vi "Single Slow IV v1.6.vi"() -> ()   [LabVIEW 2020]
uses:
  <vilib>/Utility/file.llb/Write Delimited Spreadsheet (DBL).vi
panel:
  out "DAQ_AI_Reader endpoint":refnum<k21>
  out "DAQ_CMD_Writer endpoint":refnum<k21>
  out "Current variable":dbl=2.9
  in  "stop":bool
  in  "Tab Control 2":T1(tab)=enum."PID"
  out "cRIO data plot":cluster{"Y":dbl[], "Y":dbl[]}[](graph)
  out "cRIO Plot 0":string="DC Voltage V"
  out "cRIO Plot 1":string="DC current uA"
  out "cRIO Plot 2":string="dV V"
  out "cRIO Plot 3":string="dI uA"
  out "Lockin X":cluster{"Y":dbl[], "Y":dbl[]}[](graph)
  out "Lockin Y":cluster{"Y":dbl[], "Y":dbl[]}[](graph)
  in  "Tab Control":T2(tab)
  out "Unit":string="uA"
  in  "Tab for variable":enum32{"Current", "Magnetic field"}(tab)=enum."Magnetic field"
  in  "Delay Time s":dbl=11.0 caption="Delay Time (s)"
  in  "AO Channel":string(combo)="AO0"
  in  "current output Scale factor":dbl=1.0
  in  "Fixed current uA":dbl=2.1
  in  "Scale factor":dbl=1.0
  in  "Field Rate mT per sec":dbl=0.1 format="%#_13g"
  in  "Magnet Device Select":string(combo)="NI DAQ Controlled V to I source"
  in  "Start":dbl=1.4
  in  "Range":dbl=1.5
  in  "Step":dbl=0.005
  in  "Ramp type":string(combo)="Range"
  in  "Ramp up first T":bool=TRUE
  in  "cRIO Chan 0":bool=TRUE
  in  "cRIO IP":string="//172.22.11.2"
  in  "Reading Average times":i32=20
  in  "read cRIO":bool=TRUE
  in  "Scale factor3":dbl=1.0
  in  "Channel name 3":string(combo)="dI uA"
  in  "cRIO Chan 3":bool
  in  "Scale factor2":dbl=1.0
  in  "Channel name 2":string(combo)="dV V"
  in  "cRIO Chan 2":bool
  in  "Scale factor1":dbl=1.0
  in  "Channel name 1":string(combo)="DC current uA"
  in  "cRIO Chan 1":bool=TRUE
  in  "Scale factor0":dbl=0.0001
  in  "Channel name 0":string(combo)="DC Voltage V"
  in  "Lockin address 4":string
  in  "Lockin address 3":string
  in  "Lockin address 2":string="GPIB0::9::INSTR"
  in  "Lockin address 1":string="GPIB0::8::INSTR"
  in  "Lockin 4":bool
  in  "Lockin 3":bool
  in  "Lockin 2":bool=TRUE
  in  "Lockin 1":bool=TRUE
  in  "Use Lockin":bool=TRUE
  in  "Lockin Chan name 4":string(combo)="None"
  in  "Lockin Chan name 3":string(combo)="None"
  in  "Lockin Chan name 2":string(combo)="Current mV"
  in  "Lockin Chan name 1":string(combo)="Voltage mV"
  in  "Lockin and field and temperature status":string="Data File time stamp 20210729-111405\nTemperature Chan1 1.218210, Chan2 0.050001\nmagnetic field InfmT\nLockin status\n#Device channel name Voltage mV#Device \u0000\u0000\u0000\u000fGPIB0::8::INSTR\n #PHASE=0\n #REF=1\n #FREQ=197\n #INPUT=0\n #SENS=24\n #TIMECONST=12\n #VOLTAGE=0.1\n#Device channel name Current mV#Device \u0000\u0000\u0000\u000fGPIB0::9::INSTR\n #PHASE=0\n #REF=0\n #FREQ=196.996\n #INPUT=0\n #SENS=22\n #TIMECONST=10\n #VOLTAGE=0.004\n"
  in  "Temp Device":string(combo)="Elsa"
  in  "Temp Chan1":string="T5"
  in  "Temp Chan2":string="T8"
  in  "Magnetic field read device":string(combo)="Elsa Magnet"
  in  "Record Field":bool
  in  "Contour plot folder":path=path "C:/Users/gyue/Desktop/Data folder 20210720"
  out "error out":errorcluster
  # "Voltage x factor=uA"
  # "Voltage x factor=uA"
  # "Voltage x factor=actual"
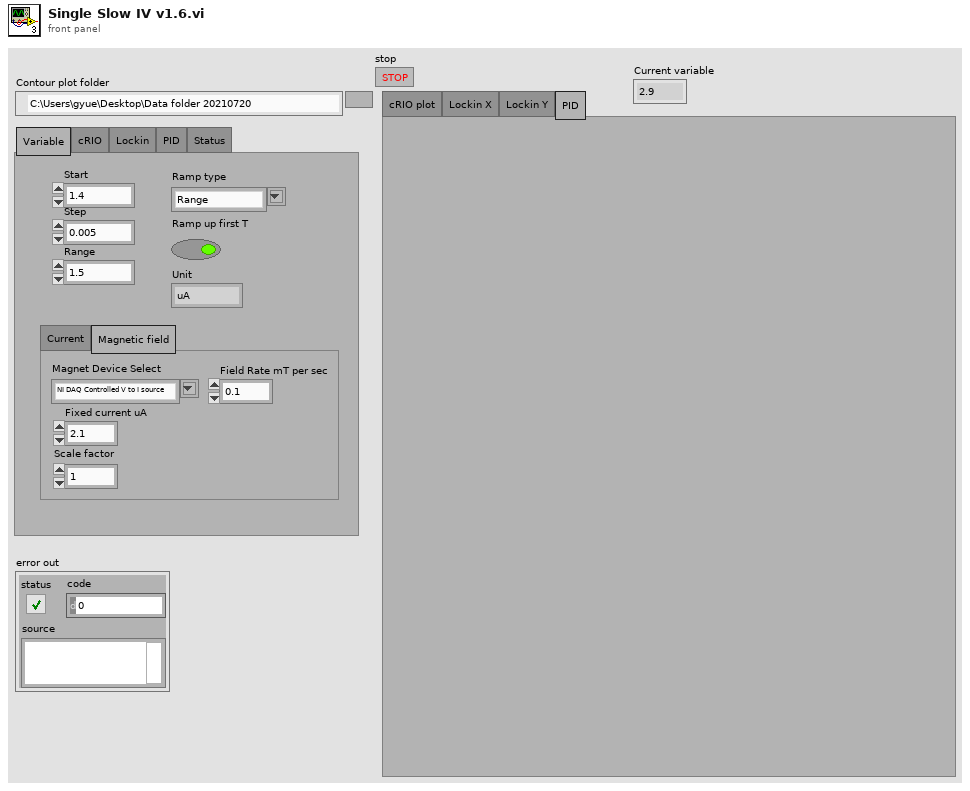
[diagram p1: front panel]
types:
  T1 = enum32{"cRIO plot", "Lockin X", "Lockin Y", "PID"}
  T2 = enum32{"Variable", "cRIO", "Lockin", "PID", "Status"}
  T3 = cluster{"AI0":dbl, "AI1":dbl, "AI2":dbl, "AI3":dbl}
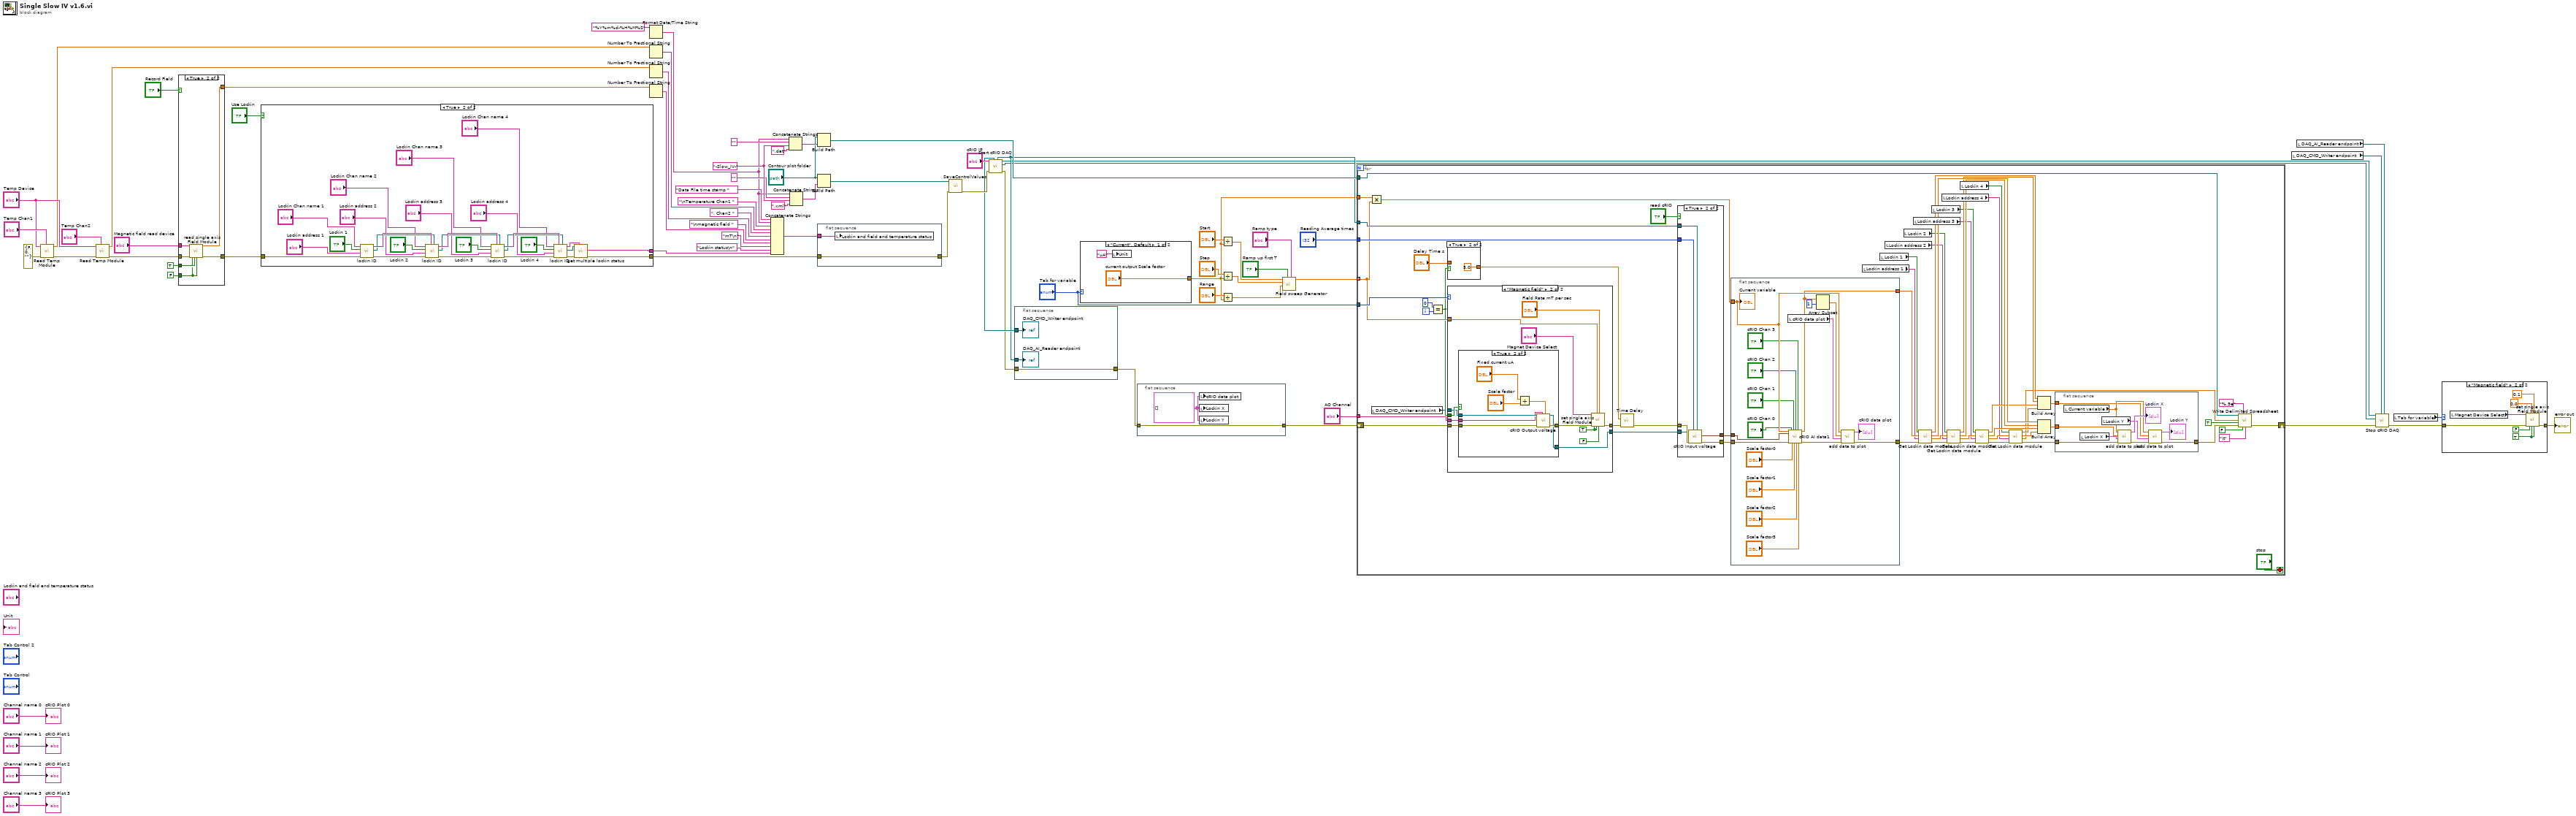
[diagram p0: block diagram]
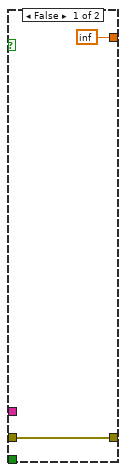
[diagram p2: hidden frame]
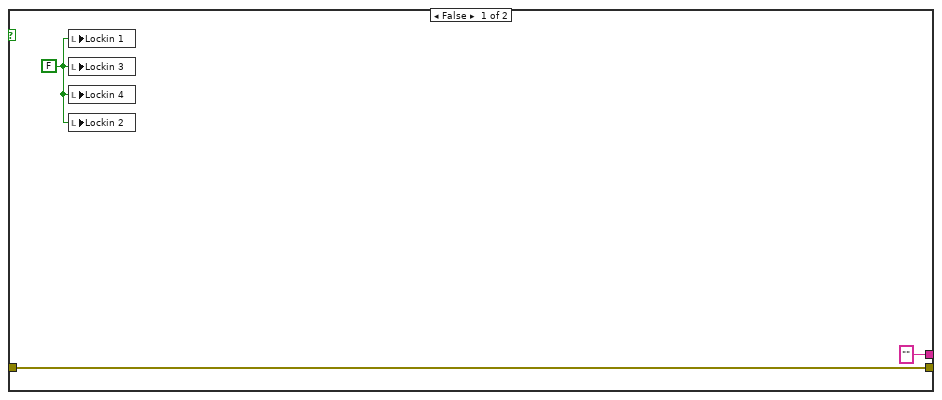
[diagram p3: hidden frame]
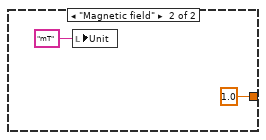
[diagram p5: hidden frame]
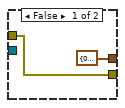
[diagram p6: hidden frame]
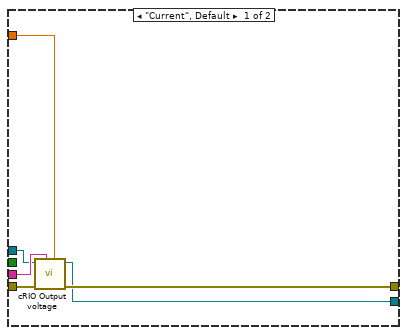
[diagram p7: hidden frame]
diagram:
  w66 = "-Slow_IV-"
  n1 = call "Read Temp Module.vi"("Temp Chan"="Temp Chan1", "error in (no error)"=errorcluster {"status"=FALSE, "code"=0, "source"=""} ("error in"), "Device"="Temp Device") -> ("error out"=w36:errorcluster, "Temperature K"=w31:dbl)  [unwired: 7 in]
  n2 = call "Read Temp Module.vi"("Temp Chan"="Temp Chan2", "error in (no error)"=w36, "Device"="Temp Device") -> ("error out"=w29:errorcluster, "Temperature K"=w30:dbl)  [unwired: 7 in]
  n3 = case shown="True" "Record Field" {
    tunnel: w29 -> [w74 w80]
    tunnel: "Magnetic field read device" -> [_ w79]
    tunnel: [inf w78] -> w27
    tunnel: TRUE ("Exec") -> [_ w77]
    tunnel: FALSE ("Init") -> [_ w76]
    tunnel: [w74 w75] -> w12
    frame False {
    }
    frame True {
      n4 = call "read single axis Field Module.vi"("Magnet Device Select"=w79, "error in (no error)"=w80, "Init"=w76, "Exec"=w77, "final"=w76) -> ("FIeld mT"=w78:dbl, "error out"=w75:errorcluster)  [unwired: 13 in]
    }
  }
  n5 = case shown="True" "Use Lockin" {
    tunnel: ["" ("Status output") w110] -> w13
    tunnel: [w83 w109] -> w11
    tunnel: w12 -> [w83 w107]
    frame False {
      w81 = FALSE ("Lockin 1")
      n6 = local write "Lockin 1"(w81) -> ()
      n7 = local write "Lockin 3"(w81) -> ()
      n8 = local write "Lockin 4"(w81) -> ()
      n9 = local write "Lockin 2"(w81) -> ()
    }
    frame True {
      n10 = call "lockin ID.vi"("error in (no error)"=w107, "Lockin address"="Lockin address 1", "Lockin on"="Lockin 1", "Lockin Chan name"="Lockin Chan name 1") -> ("error out"=w100:errorcluster, "Addresses out"=w103:refnum<visa-resource-name>[], "names out"=w104:string[])  [unwired: 5 in]
      n11 = call "lockin ID.vi"("Addresses IN"=w103, "names in"=w104, "error in (no error)"=w100, "Lockin address"="Lockin address 2", "Lockin on"="Lockin 2", "Lockin Chan name"="Lockin Chan name 2") -> ("error out"=w96:errorcluster, "Addresses out"=w97:refnum<visa-resource-name>[], "names out"=w98:string[])  [unwired: 3 in]
      n12 = call "lockin ID.vi"("Addresses IN"=w97, "names in"=w98, "error in (no error)"=w96, "Lockin address"="Lockin address 3", "Lockin on"="Lockin 3", "Lockin Chan name"="Lockin Chan name 3") -> ("error out"=w92:errorcluster, "Addresses out"=w90:refnum<visa-resource-name>[], "names out"=w91:string[])  [unwired: 3 in]
      n13 = call "lockin ID.vi"("Addresses IN"=w90, "names in"=w91, "error in (no error)"=w92, "Lockin address"="Lockin address 4", "Lockin on"="Lockin 4", "Lockin Chan name"="Lockin Chan name 4") -> ("error out"=w84:errorcluster, "Addresses out"=w85:refnum<visa-resource-name>[], "names out"=w86:string[])  [unwired: 3 in]
      n14 = call "get multiple lockin status.vi"("Device channel names"=w86, "error in (no error)"=w84, "SRS830 addresses"=w85) -> ("error out"=w109:errorcluster, "Status output"=w110:string)  [unwired: 6 in, 1 out]
    }
  }
  n15 = Format Date/Time String(time format string (%c)="%Y%m%d-%H%M%S") -> (date/time string=w23:string)  [unwired: 2 in]
  n16 = Number To Fractional String(number=w31) -> (F-format string=w20:string)  [unwired: 3 in]
  n17 = Number To Fractional String(number=w30) -> (F-format string=w19:string)  [unwired: 3 in]
  n18 = Number To Fractional String(number=w27) -> (F-format string=w17:string)  [unwired: 3 in]
  n19 = Concatenate Strings("Data File time stamp " ("string"), w23, "\nTemperature Chan1 " ("string"), w20, ", Chan2 " ("string"), w19, "\nmagnetic field " ("string"), w17, "mT\n" ("string"), "Lockin status\n" ("string"), w13) -> (w9:string)
  n20 = Concatenate Strings(w23, "" ("string"), w66, ".dat" ("string")) -> (w68:string)
  n21 = Concatenate Strings(w23, "" ("string"), w66, ".xml" ("string")) -> (w71:string)
  n22 = Build Path(base path="Contour plot folder", name or relative path=w68) -> (appended path=w53:path)
  n23 = Build Path(base path="Contour plot folder", name or relative path=w71) -> (appended path=w69:path)
  n24 = flat-sequence {
    tunnel: w11 -> [w112]
    tunnel: [w112] -> w10
    tunnel: w9 -> [w111]
    frame #0 {
      n25 = local write "Lockin and field and temperature status"(w111) -> ()
    }
  }
  n26 = call "SaveControlValues.vi"("XML File Path"=w69, "error in (no error)"=w10) -> ("error out"=w64:errorcluster)  [unwired: 8 in]
  n27 = call "Start cRIO DAQ.vi"("error in (no error)"=w64, "cRIO IP"="cRIO IP") -> ("error out"=w4:errorcluster, "vi reference"=w1:refnum<vi>, "application reference"=w2:refnum<vi>, "DAQ_AI_Reader endpoint"=w51:refnum<k21>, "DAQ_CMD_Writer endpoint"=w52:refnum<k21>)  [unwired: 5 in]
  n28 = flat-sequence {
    tunnel: w52 -> [w115]
    tunnel: w51 -> [w114]
    tunnel: w4 -> [w113]
    tunnel: [w113] -> w3
    frame #0 {
      "DAQ_CMD_Writer endpoint" <- w115
      "DAQ_AI_Reader endpoint" <- w114
    }
  }
  n29 = case shown="\"Current\", Default" "Tab for variable" {
    tunnel: ["current output Scale factor" 1.0 ("current output Scale factor")] -> w40
    frame "Current", Default {
      n30 = local write "Unit"("uA" ("Unit")) -> ()
    }
    frame "Magnetic field" {
      n31 = local write "Unit"("mT" ("Unit")) -> ()
    }
  }
  n32 = flat-sequence {
    tunnel: w3 -> [w121]
    tunnel: [w121] -> w7
    frame #0 {
      w120 = cluster{dbl[], dbl[]}[] [] ("appended array")
      n33 = local write "cRIO data plot"(w120) -> ()
      n34 = local write "Lockin X"(w120) -> ()
      n35 = local write "Lockin Y"(w120) -> ()
    }
  }
  n36 = Divide(x="Start", y=w40) -> (x/y=w42:dbl)
  n37 = Divide(x="Step", y=w40) -> (x/y=w57:dbl)
  n38 = Divide(x="Range", y=w40) -> (x/y=w56:dbl)
  n39 = call "Field sweep Generator.vi"("Ramp type"="Ramp type", "Ramp up first T"="Ramp up first T", "Field Radius"=w56, "Field step"=w57, "Field Origin"=w42) -> ("output array"=w54:dbl[])  [unwired: 6 in]
  n40 = for {
    tunnel: "AO Channel" -> [w161]
    tunnel: w54 -> [w162] mode=indexing
    tunnel: w51 -> [w177]
    tunnel: w53 -> [w176]
    tunnel: "Reading Average times" -> [w169]
    tunnel: "Tab for variable" -> [w163]
    tunnel: w40 -> [w157]
    shift-right: [w170] -> w48
    shift-left: w7 -> [w155]
    i -> [w167]
    stop <- "stop" stop-if-true
    n41 = Multiply(x=w157, y=w162) -> (x*y=w153:dbl)
    n42 = local read "DAQ_CMD_Writer endpoint"() -> (w122:refnum<k21>)
    n43 = Equal?(x=0, y=w167) -> (x = y?=w158:bool)
    n44 = case shown="True" w158 {
      tunnel: "Delay Time s" -> [w242 _]
      tunnel: [w242 5.0 ("Delay Time s")] -> w164
      frame False {
      }
      frame True {
      }
    }
    n45 = case shown="\"Magnetic field\"" w163 {
      tunnel: w162 -> [w219 w223]
      tunnel: w161 -> [w218 w227]
      tunnel: w155 -> [w217 w230]
      tunnel: w122 -> [w216 w229]
      tunnel: [w215 w225] -> w160
      tunnel: [w214 w228] -> w159
      tunnel: w158 -> [_ w231]
      frame "Current", Default {
        n46 = call "cRIO Output voltage.vi"("Voltage"=w219, "AO Channel"=w218, "error in (no error)"=w217, "DAQ_CMD_Writer endpoint"=w216) -> ("error out"=w215:errorcluster, "DAQ_CMD_Writer endpoint out"=w214:refnum<k21>)  [unwired: 6 in]
      }
      frame "Magnetic field" {
        w221 = TRUE ("Init")
        n47 = case shown="True" w231 {
          tunnel: w230 -> [w232 w241]
          tunnel: [w232 w240] -> w226
          tunnel: w229 -> [w233 w239]
          tunnel: [w233 w238] -> w228
          tunnel: w227 -> [_ w237]
          frame False {
          }
          frame True {
            n48 = Divide(x="Fixed current uA", y="Scale factor") -> (x/y=w235:dbl)
            n49 = call "cRIO Output voltage.vi"("Voltage"=w235, "AO Channel"=w237, "error in (no error)"=w241, "DAQ_CMD_Writer endpoint"=w239) -> ("error out"=w240:errorcluster, "DAQ_CMD_Writer endpoint out"=w238:refnum<k21>)  [unwired: 6 in]
          }
        }
        n50 = call "set single axis Field Module.vi"("Magnet Device Select"="Magnet Device Select", "error in (no error)"=w226, "Init"=w221, "Field Target mT"=w223, "Exec"=w221, "Field Rate mT per sec"="Field Rate mT per sec", "final"=FALSE ("Exec")) -> ("error out"=w225:errorcluster)  [unwired: 12 in]
      }
    }
    n51 = call "Time Delay"("error in (no error)"=w160, "Delay Time (s)"=w164) -> ("error out"=w172:errorcluster)  [unwired: 9 in]
    n52 = case shown="True" "read cRIO" {
      tunnel: w177 -> [_ w213]
      tunnel: w172 -> [w207 w212]
      tunnel: [w207 w211] -> w151
      tunnel: w169 -> [_ w210]
      tunnel: w159 -> [_ w209]
      tunnel: [T3 {"AI0"=0.0, "AI1"=0.0, "AI2"=0.0, "AI3"=0.0} ("output cluster") w208] -> w152
      frame False {
      }
      frame True {
        n53 = call "cRIO Input voltage.vi"("DAQ_AI_Reader endpoint"=w213, "Average"=w210, "error in (no error)"=w212, "DAQ_CMD_Writer endpoint"=w209) -> ("error out"=w211:errorcluster, "output cluster"=w208:T3)  [unwired: 5 in, 1 out]
      }
    }
    n54 = flat-sequence {
      tunnel: w153 -> [w204]
      tunnel: w152 -> [w203]
      tunnel: w151 -> [w202]
      tunnel: [w195] -> w150
      tunnel: [w190] -> w149
      frame #0 {
        n55 = local read "cRIO data plot"() -> (w205:cluster{"Y":dbl[], "Y":dbl[]}[])
        n56 = call "cRIO AI data1.vi"("I"=w204, "Input cluster"=w203, "error in (no error)"=w202, "Chan 0"="cRIO Chan 0", "Scale factor0"="Scale factor0", "Chan 1"="cRIO Chan 1", "Scale factor1"="Scale factor1", "Chan 2"="cRIO Chan 2", "Scale factor2"="Scale factor2", "Chan 3"="cRIO Chan 3", "Scale factor3"="Scale factor3") -> ("Output data"=w190:dbl[], "error out"=w196:errorcluster)  [unwired: 7 in]
        n57 = Array Subset(array=w190, index=1) -> (w188:dbl[])  [unwired: 1 in]
        n58 = call "add data to plot.vi"("error in (no error)"=w196, "Input graph"=w205, "Input Y array"=w188, "x"=w204) -> ("error in (no error) 2"=w195:errorcluster, "Output graph"=→"cRIO data plot":cluster{dbl[], dbl[]}[])  [unwired: 6 in]
        "Current variable" <- w204
      }
    }
    n59 = local read "Lockin address 1"() -> (w143:string)
    n60 = local read "Lockin 1"() -> (w154:bool)
    n61 = local read "Lockin address 2"() -> (w140:string)
    n62 = local read "Lockin 2"() -> (w142:bool)
    n63 = local read "Lockin address 3"() -> (w133:string)
    n64 = call "Get Lockin data module.vi"("error in (no error)"=w150, "Lockin address 1"=w143, "Output data in"=w149, "Lockin 1"=w154) -> ("error out"=w139:errorcluster, "Output data out"=w141:dbl[], "X mV"=w147:dbl, "Y mV"=w145:dbl)  [unwired: 4 in]
    n65 = local read "Lockin 3"() -> (w136:bool)
    n66 = local read "Lockin address 4"() -> (w127:string)
    n67 = call "Get Lockin data module.vi"("error in (no error)"=w139, "Lockin address 1"=w140, "Output data in"=w141, "Lockin 1"=w142) -> ("error out"=w134:errorcluster, "Output data out"=w135:dbl[], "X mV"=w137:dbl, "Y mV"=w138:dbl)  [unwired: 4 in]
    n68 = local read "Lockin 4"() -> (w130:bool)
    n69 = call "Get Lockin data module.vi"("error in (no error)"=w134, "Lockin address 1"=w133, "Output data in"=w135, "Lockin 1"=w136) -> ("error out"=w128:errorcluster, "Output data out"=w129:dbl[], "X mV"=w131:dbl, "Y mV"=w132:dbl)  [unwired: 4 in]
    n70 = call "Get Lockin data module.vi"("error in (no error)"=w128, "Lockin address 1"=w127, "Output data in"=w129, "Lockin 1"=w130) -> ("error out"=w124:errorcluster, "Output data out"=w123:dbl[], "X mV"=w125:dbl, "Y mV"=w126:dbl)  [unwired: 4 in]
    n71 = Build Array(w145, w138, w132, w126) -> (w144:dbl[])
    n72 = Build Array(w147, w137, w131, w125) -> (w146:dbl[])
    n73 = flat-sequence {
      tunnel: w124 -> [w184]
      tunnel: [w182] -> w148
      tunnel: w146 -> [w185]
      tunnel: w144 -> [w178]
      frame #0 {
        n74 = local read "Current variable"() -> (w181:dbl)
        n75 = local read "Lockin X"() -> (w187:cluster{"Y":dbl[], "Y":dbl[]}[])
        n76 = local read "Lockin Y"() -> (w180:cluster{"Y":dbl[], "Y":dbl[]}[])
        n77 = call "add data to plot.vi"("error in (no error)"=w184, "Input graph"=w187, "Input Y array"=w185, "x"=w181) -> ("error in (no error) 2"=w183:errorcluster, "Output graph"=→"Lockin X":cluster{dbl[], dbl[]}[])  [unwired: 6 in]
        n78 = call "add data to plot.vi"("error in (no error)"=w183, "Input graph"=w180, "Input Y array"=w178, "x"=w181) -> ("error in (no error) 2"=w182:errorcluster, "Output graph"=→"Lockin Y":cluster{dbl[], dbl[]}[])  [unwired: 6 in]
      }
    }
    n79 = call-poly <vilib>:"Write Delimited Spreadsheet.vi"("file path (dialog if empty)"=w176, "format (%.3f)"="%.9e", "1D data"=w123, "append to file? (new file:F)"=TRUE, "error in (no error)"=w148, "transpose? (no:F)"=FALSE, "delimiter (\\t)"="\t" ("delimiter (\\t)")) -> ("error out"=w170:errorcluster)  [unwired: 7 in, 1 out]
  }
  n80 = local read "DAQ_CMD_Writer endpoint"() -> (w6:refnum<k21>)
  n81 = local read "DAQ_AI_Reader endpoint"() -> (w5:refnum<k21>)
  n82 = call "Stop cRIO DAQ.vi"("DAQ_AI_Reader endpoint"=w5, "DAQ_CMD_Writer endpoint"=w6, "error in (no error)"=w48, "VI reference"=w1, "application reference"=w2) -> ("error out"=w38:errorcluster)  [unwired: 6 in]
  n83 = local read "Tab for variable"() -> (w39:enum32{"Current", "Magnetic field"})
  n84 = case shown="\"Magnetic field\"" w39 {
    tunnel: w38 -> [w244 w248]
    tunnel: [w244 w247] -> w37
    frame "Current", Default {
    }
    frame "Magnetic field" {
      w245 = TRUE ("Exec")
      n85 = local read "Magnet Device Select"() -> (w251:string)
      n86 = call "set single axis Field Module.vi"("Magnet Device Select"=w251, "error in (no error)"=w248, "Init"=FALSE, "Field Target mT"=0.0, "Exec"=w245, "Field Rate mT per sec"=0.1, "final"=w245) -> ("error out"=w247:errorcluster)  [unwired: 12 in]
    }
  }
  "error out" <- w37
  "cRIO Plot 0" <- "Channel name 0"
  "cRIO Plot 1" <- "Channel name 1"
  "cRIO Plot 2" <- "Channel name 2"
  "cRIO Plot 3" <- "Channel name 3"
